vi "monocromActon.vi"(9 "Lamda":dbl, 11 "VISA resource name":refnum<visa-resource-name>="COM3") -> (1 "Sal:Lamda":dbl)   [LabVIEW 2016]
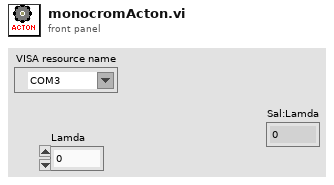
[diagram p1: front panel]
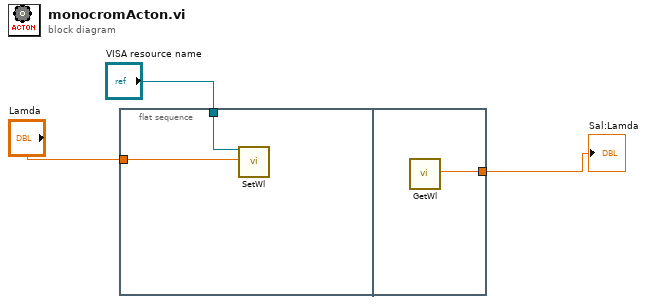
[diagram p0: block diagram]
diagram:
  n1 = flat-sequence {
    tunnel: "VISA resource name" -> [w5]
    tunnel: "Lamda" -> [w4]
    tunnel: [w6] -> w1
    frame #0 {
      n2 = call "SetWl.vi"("VISA resource name"=w5, "Wavelength (nm)"=w4) -> ()  [unwired: 16 in, 2 out]
    }
    frame #1 {
      n3 = call "GetWl.vi"() -> ("Wavelength"=w6:dbl)  [unwired: 17 in, 2 out]
    }
  }
  "Sal:Lamda" <- w1
